vi "Run TSA Project.vi"(7 "Silent Mode? (T)":bool=TRUE, 8 "error in (no error)":errorcluster, 9 "Report Path (Optional)":path, 10 "TestStand Bin Directory":path=path "C:/Program Files (x86)/National Instruments/TestStand 2019/Bin", 11 "TestStand Sequence Analyzer Project":path) -> (0 "error out":errorcluster, 1 "TSA Messages as Plain Text":string, 2 "TSA Messages[]":T1[](array[typedef]), 3 "No Errors?":bool)   [LabVIEW 2016, in "SLL TestStand.lvlib"]
doc: "Runs a TestStand Sequence Analyzer Project and returns if there are any errors.\n\nhttps://zone.ni.com/reference/en-XX/help/370052AA-01/tsref/infotopics/sequence_analyzer/"
uses:
  SLL TestStand.lvlib
  _Typedefs/TSA Error Message Cluster.ctl
  SLL File IO/SLL File IO.lvlib
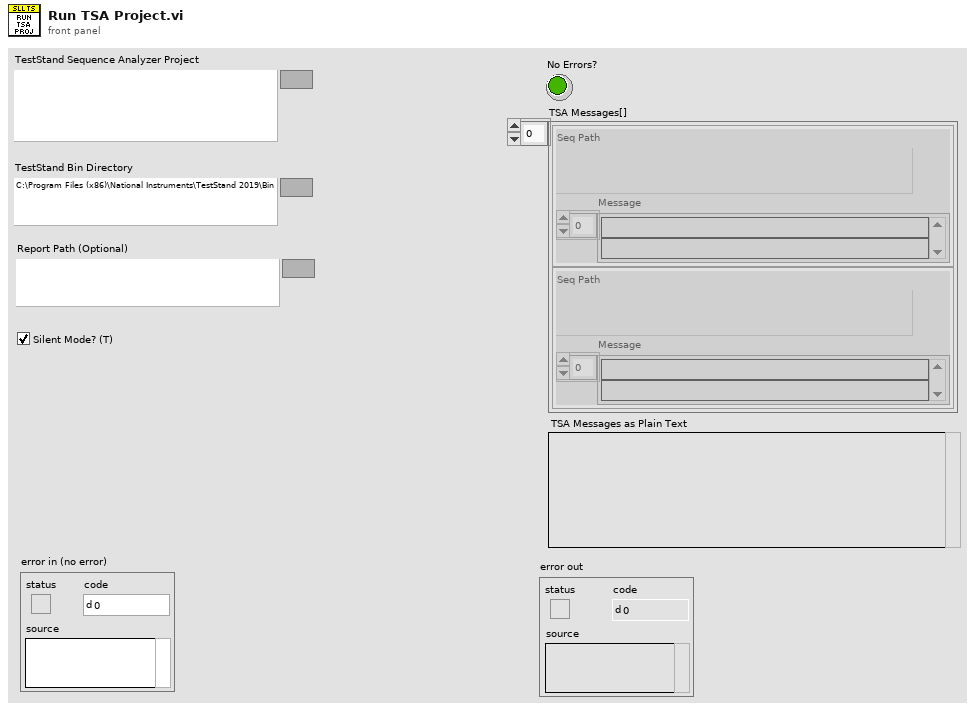
[diagram p1: front panel]
types:
  T1 = typedef "SLL TestStand.lvlib/TSA Error Message Cluster.ctl" = cluster{"Seq Path":path, "Message":string[]}
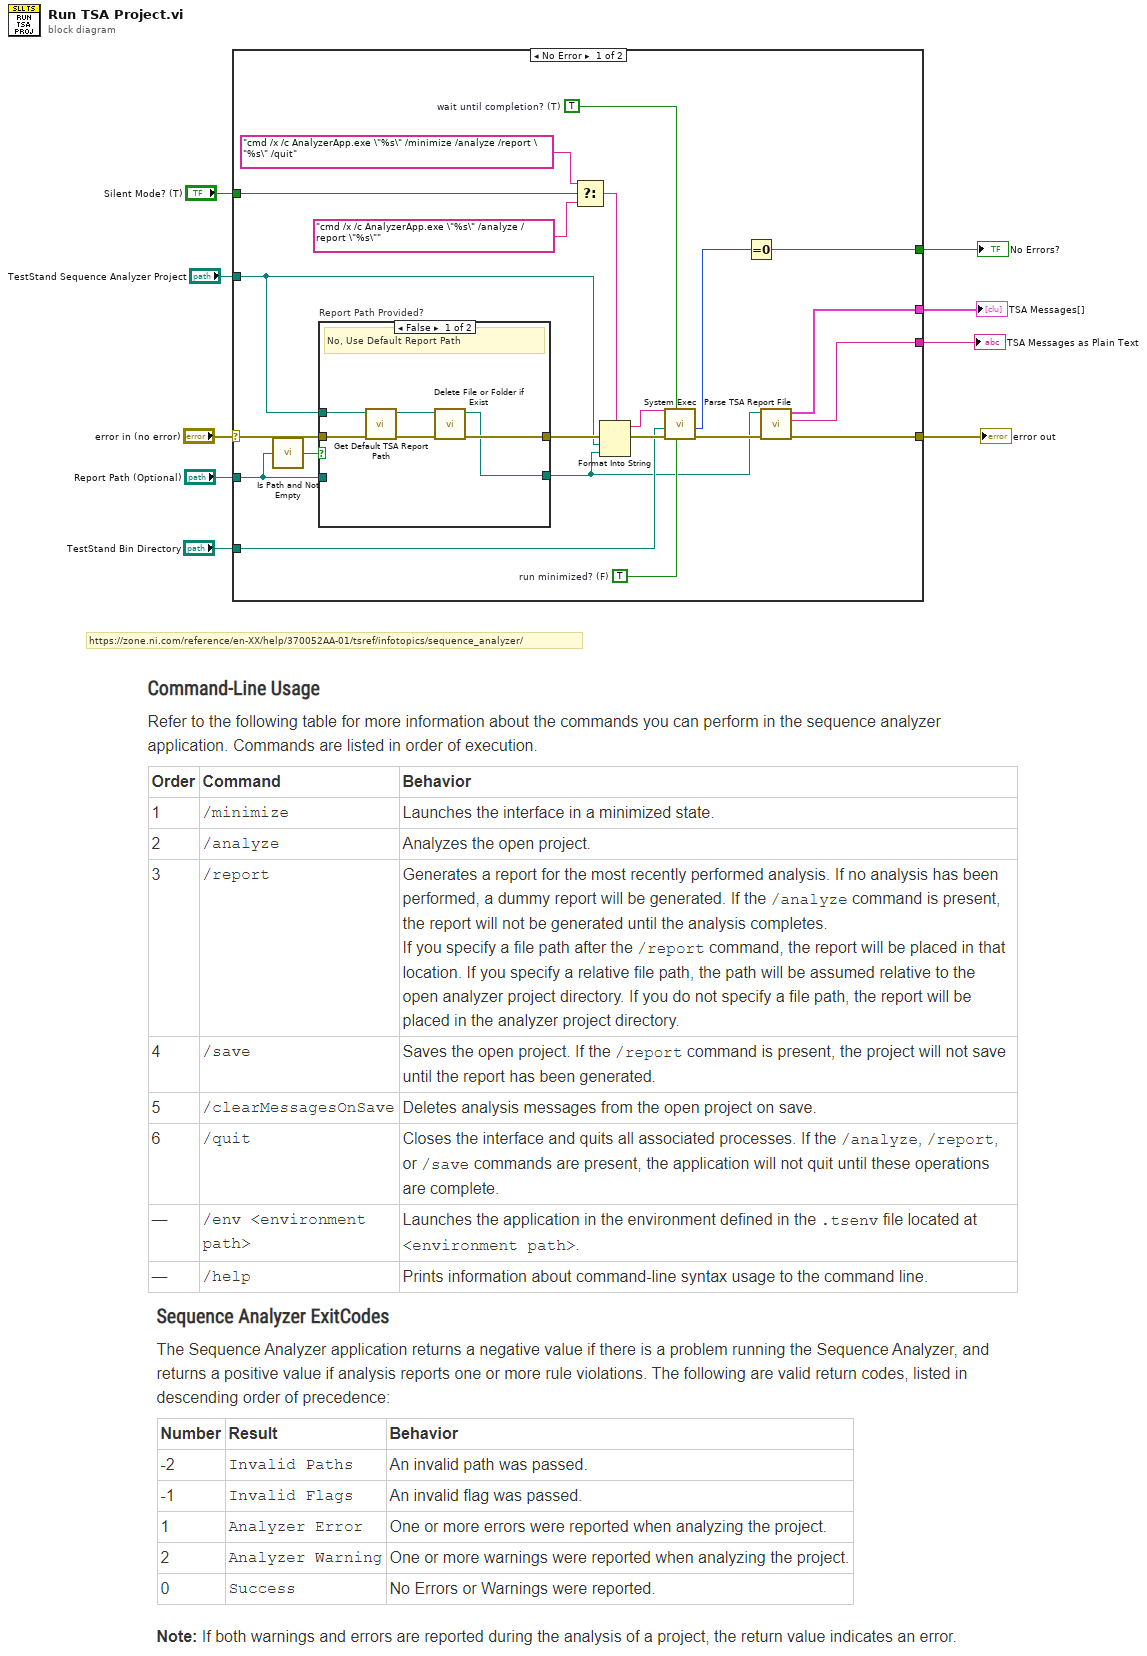
[diagram p0: block diagram]
diagram:
  # "https://zone.ni.com/reference/en-XX/help/370052AA-01/tsref/infotopics/sequence_analyzer/"
  n1 = case shown="No Error" "error in (no error)" {
    selector: "error in (no error)" -> [w30 w39]
    tunnel: [w13 w39] -> w8
    tunnel: "TestStand Sequence Analyzer Project" -> [w15 _]
    tunnel: "TestStand Bin Directory" -> [w27 _]
    tunnel: [w23 _] -> w5
    tunnel: "Silent Mode? (T)" -> [w21 _]
    tunnel: "Report Path (Optional)" -> [w14 _]
    tunnel: [w11 _] -> w2
    tunnel: [w10 _] -> w1
    frame No Error {
      w22 = TRUE  # run minimized? (F)
      w25 = TRUE  # wait until completion? (T)
      n2 = call <vilib>:"Is Path and Not Empty.vi"("path"=w14) -> ("Is Path and Not Empty?"=w16:bool)  [unwired: 4 in]
      n3 = case "Report Path Provided?" shown="False" w16 {
        tunnel: w30 -> [w36 w37]
        tunnel: [w33 w37] -> w17
        tunnel: w15 -> [w34 _]
        tunnel: [w31 w38] -> w12
        tunnel: w14 -> [_ w38]
        frame False {
          # "No, Use Default Report Path"
          n4 = call "Get Default TSA Report Path.vi"("error in (no error)"=w36, "TestStand Sequence Analyzer Project"=w34) -> ("error out"=w35:errorcluster, "TSA Report Path"=w32:path)  [unwired: 8 in]
          n5 = call "Delete File or Folder if Exist.vi"("error in (no error)"=w35, "Path"=w32) -> ("error out"=w33:errorcluster, "Path out"=w31:path)  [unwired: 8 in]
        }
        frame True {
          # "Yes"
        }
      }
      n6 = Select(t="cmd /x /c AnalyzerApp.exe \"%s\" /minimize /analyze /report \"%s\" /quit" ("command line"), s=w21, f="cmd /x /c AnalyzerApp.exe \"%s\" /analyze /report \"%s\"" ("command line")) -> (s? t:f=w19:string)
      n7 = Format Into String(format string=w19, error in=w17, w15, w12) -> (resulting string=w26:string, error out=w28:errorcluster)  [unwired: 1 in]
      n8 = call <vilib>:"System Exec.vi"("run minimized? (F)"=w22, "wait until completion? (T)"=w25, "error in (no error)"=w28, "working directory"=w27, "command line"=w26) -> ("error out"=w29:errorcluster, "return code"=w24:i32)  [unwired: 3 in, 2 out]
      n9 = Equal To 0?(x=w24) -> (x = 0?=w23:bool)
      n10 = call "Parse TSA Report File.vi"("error in (no error)"=w29, "TSA Report File Path"=w12) -> ("error out"=w13:errorcluster, "TSA Errors as Plain Text"=w10:string, "TSA Messages[]"=w11:T1[])  [unwired: 7 in]
    }
    frame Error {
    }
  }
  "error out" <- w8
  "No Errors?" <- w5
  "TSA Messages[]" <- w2
  "TSA Messages as Plain Text" <- w1
